vi "host_main(deprecated).vi"() -> ()   [LabVIEW 2023]
uses:
  JSON Command.ctl
  Action.ctl
  <vilib>/FPGAPlugInAG/cRIO-9048/niLvFpga_Open_cRIO-9048.vi
  <vilib>/rvi/interface/common/dynamic/niFpgaDynamicAddResources.vi
  <vilib>/Utility/error.llb/Error Cluster From Error Code.vi
  <vilib>/rvi/errors/niLvFpgaAdjustHostInterfaceError.vi
  <vilib>/rvi/interface/common/niFpgaWaitOnOcc.vi
  <vilib>/FPGAPlugInAG/Dynamic/niLvFpga_Run_Dynamic.vi
  <vilib>/FPGAPlugInAG/Dynamic/niLvFpga_Close_Dynamic.vi
  <vilib>/rvi/interface/nirviOpenFPGA/nirviOpenFPGA.xnode
  FPGA Bitfiles/fpgaproj_FPGATarget_targetmainmem_EQ1ZdgFzOzw.lvbitx
  target_main_mem.vi
  <vilib>/rvi/interface/nirviReadWriteControl/nirviReadWriteControl.xnode
  <vilib>/rvi/interface/nirviMethod/nirviMethod.xnode
  <vilib>/rvi/interface/nirviCloseFPGA/nirviCloseFPGA.xnode
  <vilib>/FPGAPlugInAG/Dynamic/niLvFpga_ConfigureFifo_Dynamic.vi
  <vilib>/rvi/errors/niLvFpgaMergeErrorWithErrorCode.vi
  <vilib>/FPGAPlugInAG/Dynamic/niLvFpga_WriteFifo_Dynamic.vi
  NiFpgaLv.dll
  <vilib>/rvi/interface/Simulation/niFpgaSimulationCallBeginRW.vi
  <vilib>/FPGAPlugInAG/Dynamic/niLvFpga_ReadFifo_Dynamic.vi
  <vilib>/FPGAPlugInAG/Dynamic/niLvFpga_StopFifo_Dynamic.vi
panel:
  out "bytes written":i32
  in  "Stop VI":bool
  out "FPGA VI Reference Out":refnum<k20>
  out "Abort":bool
  out "remote port":u16
  out "remote address":string
  in  "Send PORT":u16=7704
  out "From Client:":string
  out "RAW JSON":T1
  out "ACK sent":string
  out "Laser Toggle 2":bool
  out "Laser Toggle 1":bool
  out "Laser Toggle 0":bool
  in  "Analogue Line 5":u32=10
  in  "Analogue Line 4":u32=10
  in  "Analogue Line 3":u32=10
  out "Digital Line 2":u32
  out "Digital Line 1":u32
  out "Digital Line 0":u32
  out "Analogue Line 2":u8
  out "Analogue Line 1":u8
  out "Analogue Line 0":u8
  in  "FPGA Status Update Loop Time (ms)":u32=1
  out "UDP Sent":string
  in  "Event":string
  in  "Status":string
  in  "Receive PORT":u16=7705
  in  "UDP Address (IP)":string="172.22.11.1"
  out "Boolean array on Host":bool[](array[boolean])
  out "Addr Digital 2":u32
  out "Addr Digital 1":u32
  out "Addr Analogue 1":u32
  out "Addr Analogue 2":u32
  out "Addr Digital 0":u32
  out "Addr Analogue 0":u32
  in  "Digital 2 Action Table":T2[](array[typedef])
  in  "Digital 1 Action Table":T2[](array[typedef])
  in  "Digital 0 Action Table":T2[](array[typedef])
  in  "Analogue 2 Action Table":T2[](array[typedef])
  in  "Analogue 1 Action Table":T2[](array[typedef])
  in  "Analogue 0 Action Table":T2[](array[typedef])
  # "TCP Communication"
  # "Angle, Phase, and Color"
  # "UDP Communication"
  # "Laser On/Off and Power Control"
  # "Action Tables & Experiment Logging"
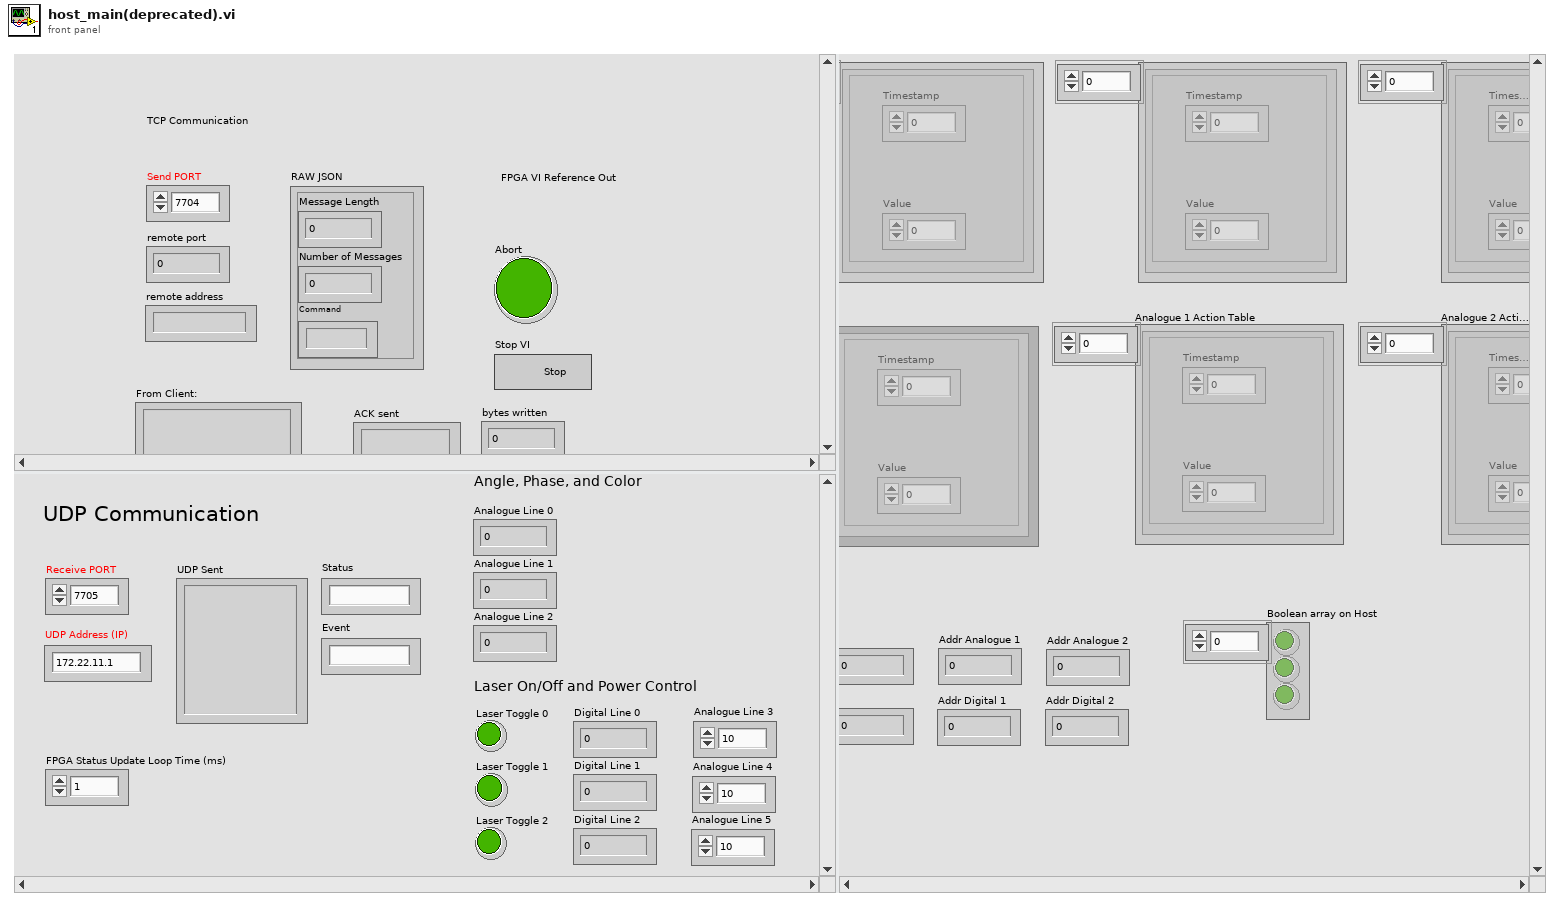
[diagram p1: front panel]
types:
  T1 = typedef "JSON Command.ctl" = cluster{"Message Length":i32, "Number of Messages":i32, "Command":string}
  T2 = typedef "Action.ctl" = cluster{"Timestamp":u32, "Value":u32}
  T3 = cluster{"Digital 2":bool, "Digital 1":bool, "Digital 0":bool}
  T4 = cluster{"Digitals":u8, "Analogue 0":u8, "Analogue 1":u8, "Event":string, "Analogue 2":u8, "Analogue 3":u32, "Analogue 4":u32, "Analogue 5":u32}
  T5 = enum16{"Standard", "Buffered", "CRLF", "Immediate"}
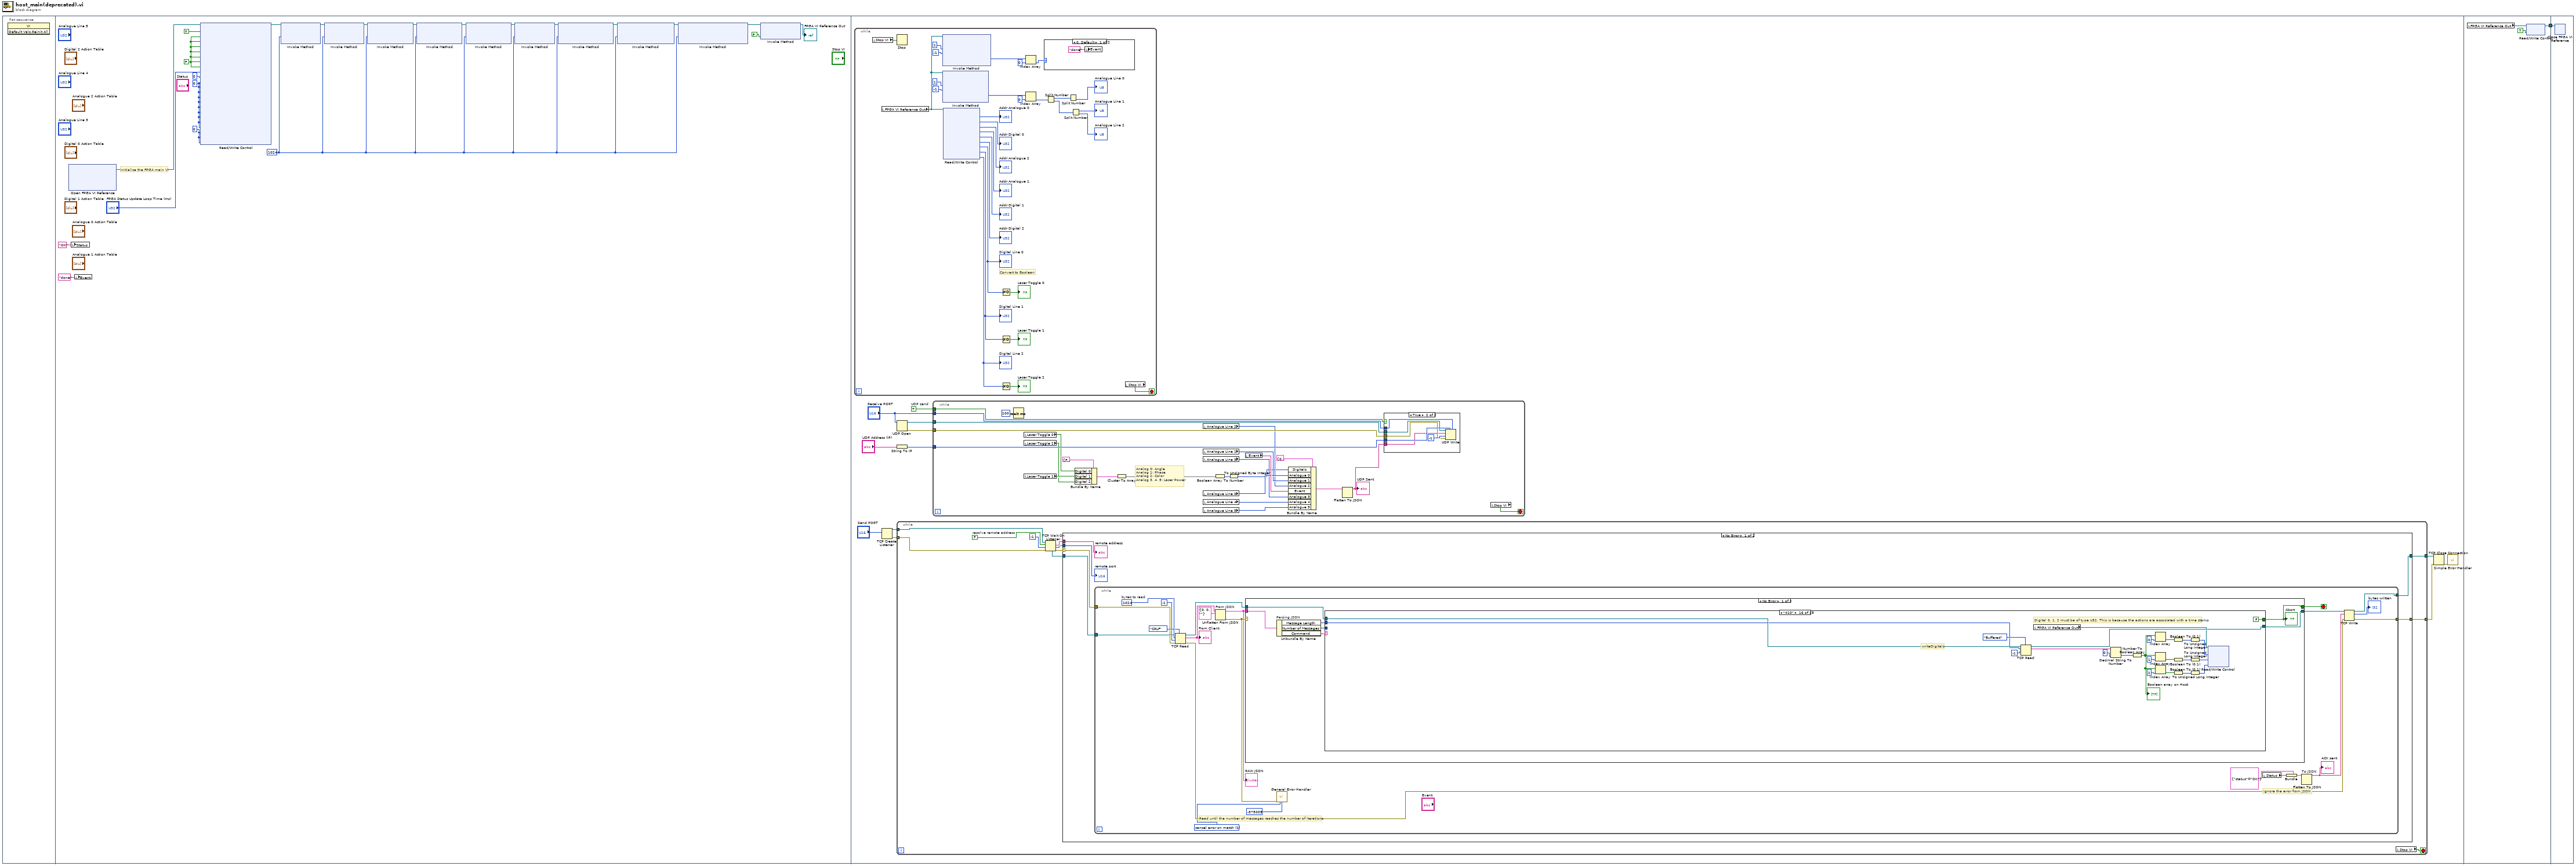
[diagram p0: block diagram]
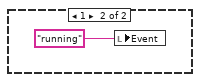
[diagram p2: hidden frame]
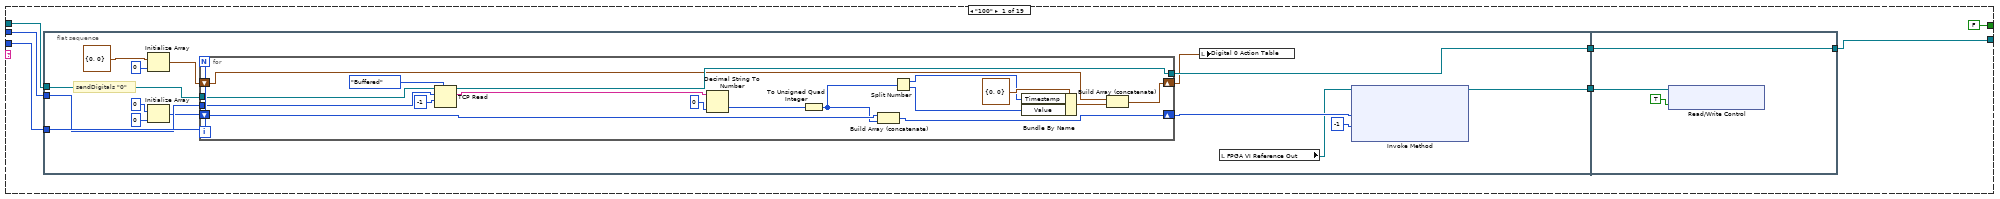
[diagram p4: hidden frame]
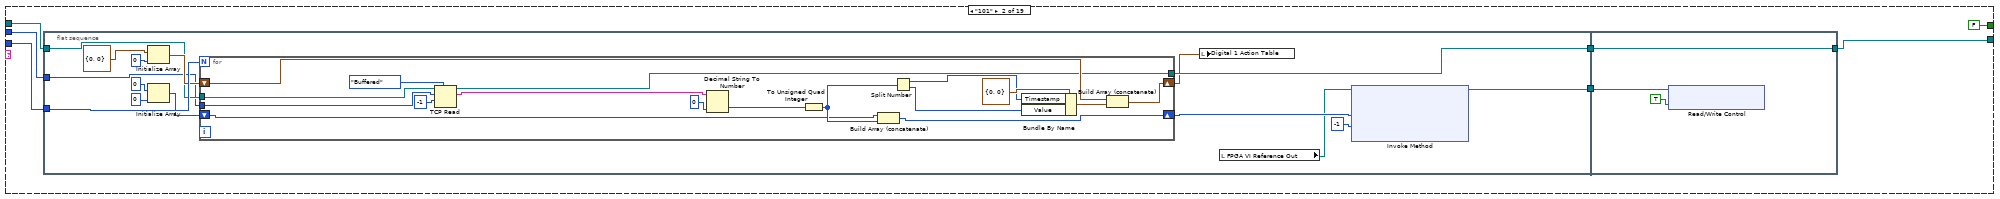
[diagram p5: hidden frame]
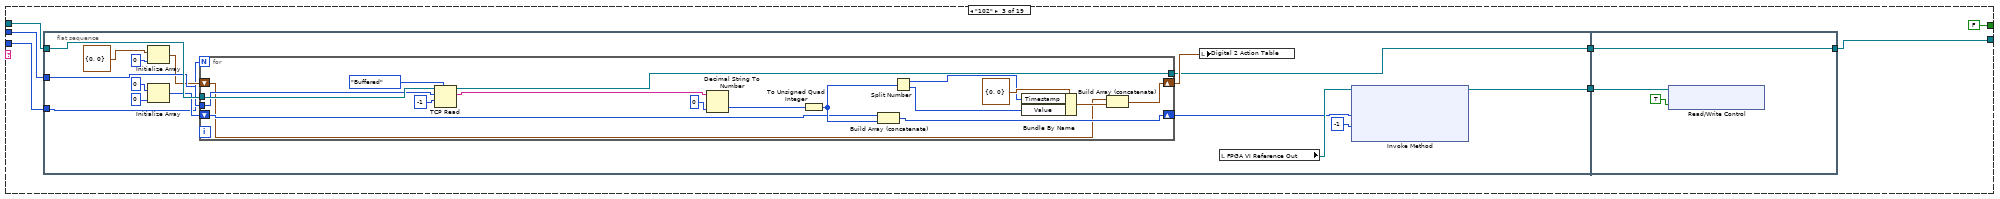
[diagram p6: hidden frame]
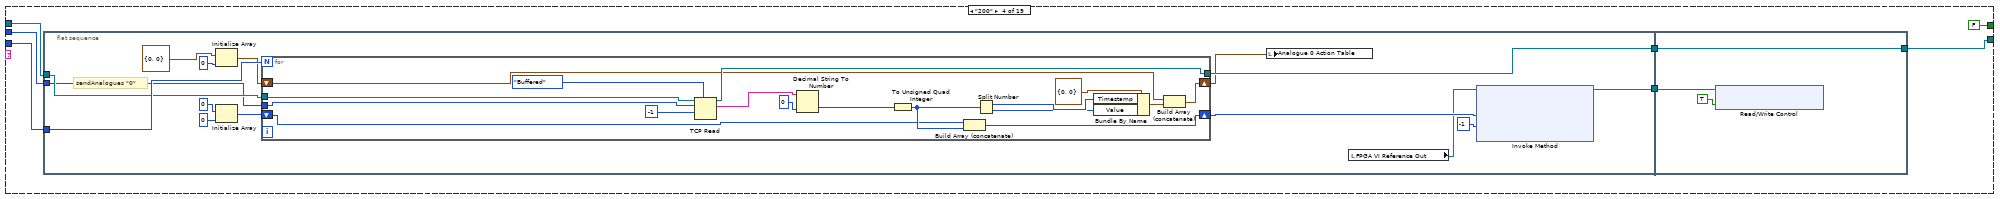
[diagram p7: hidden frame]
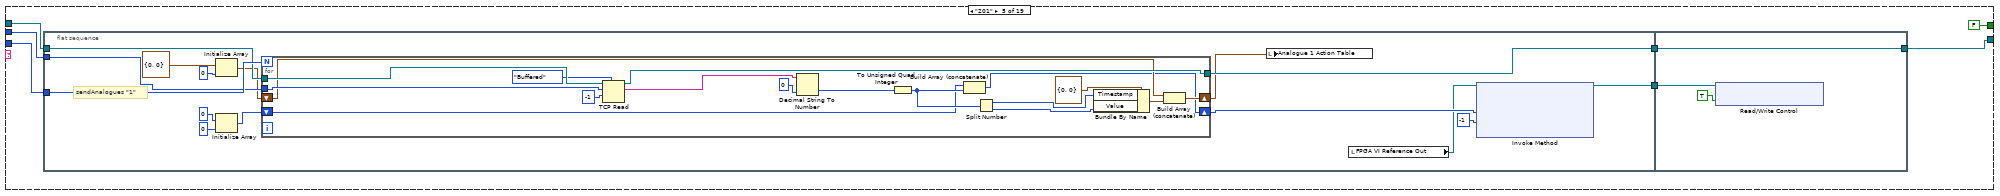
[diagram p8: hidden frame]
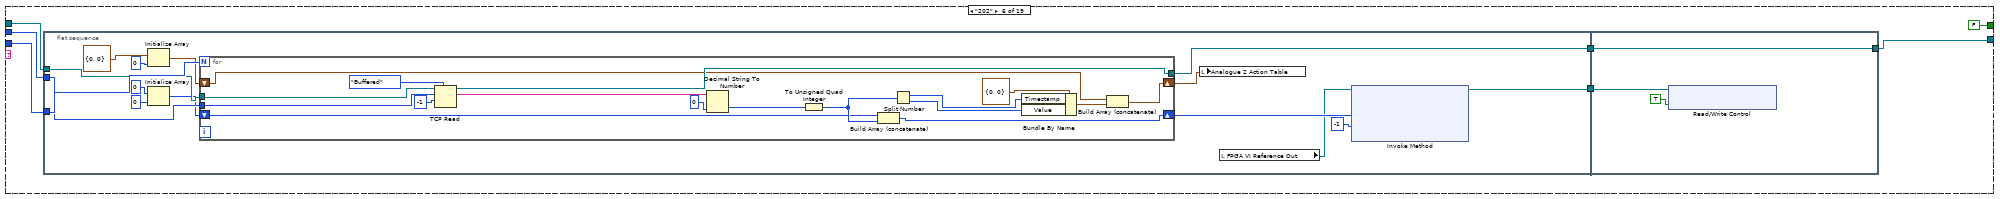
[diagram p9: hidden frame]
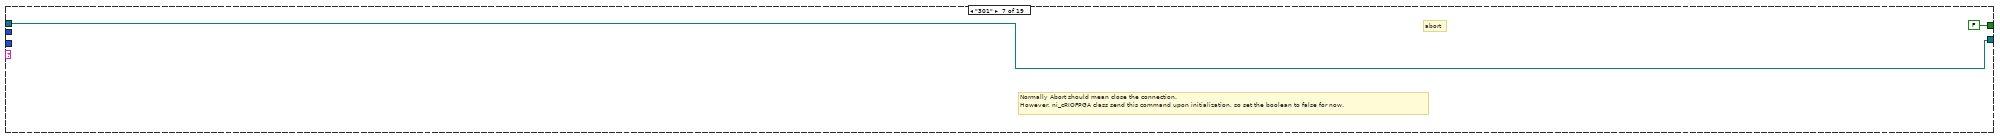
[diagram p10: hidden frame]
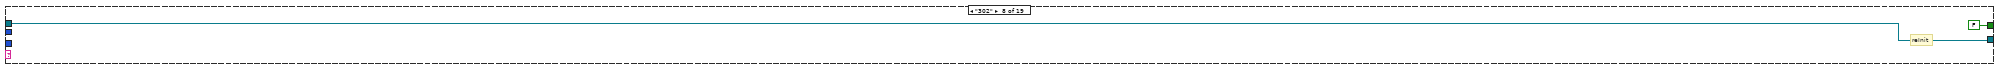
[diagram p11: hidden frame]
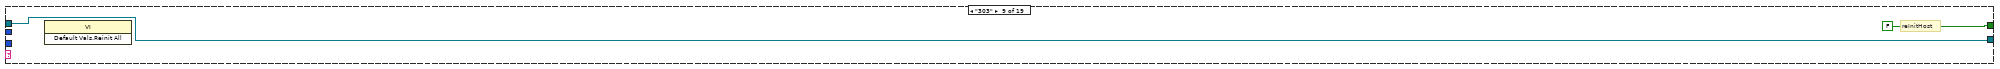
[diagram p12: hidden frame]
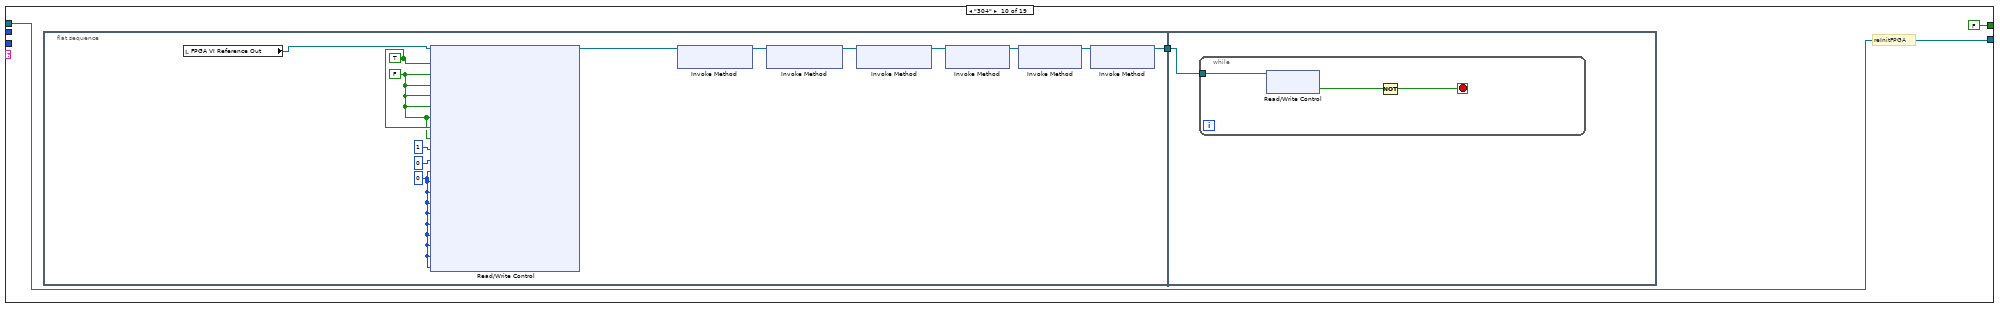
[diagram p13: hidden frame]
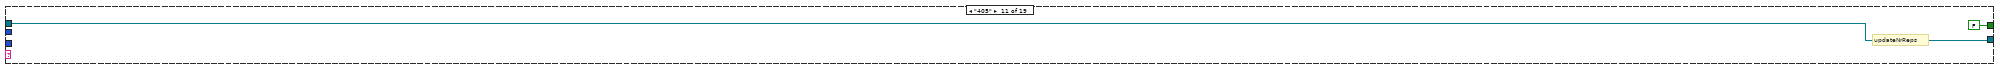
[diagram p14: hidden frame]
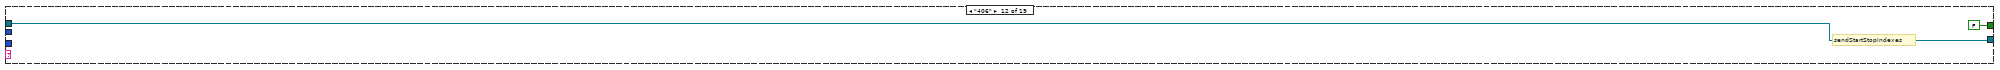
[diagram p15: hidden frame]
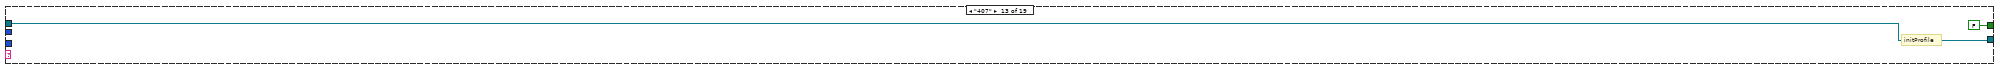
[diagram p16: hidden frame]
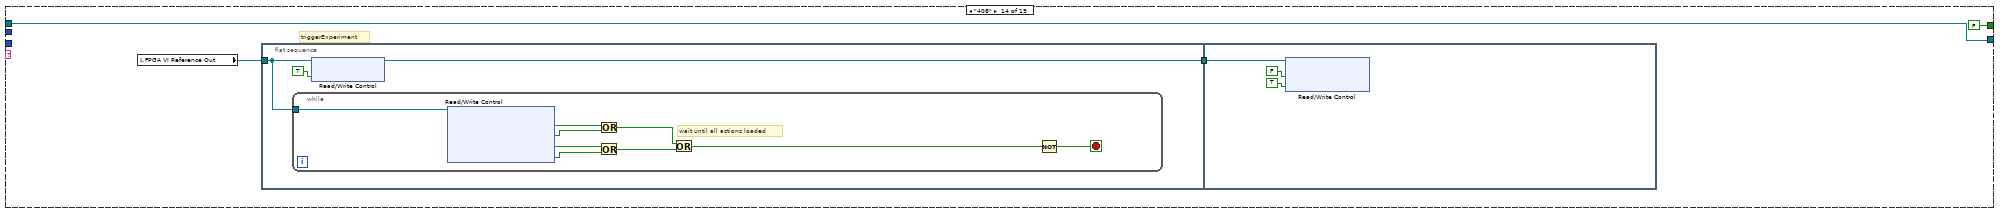
[diagram p17: hidden frame]
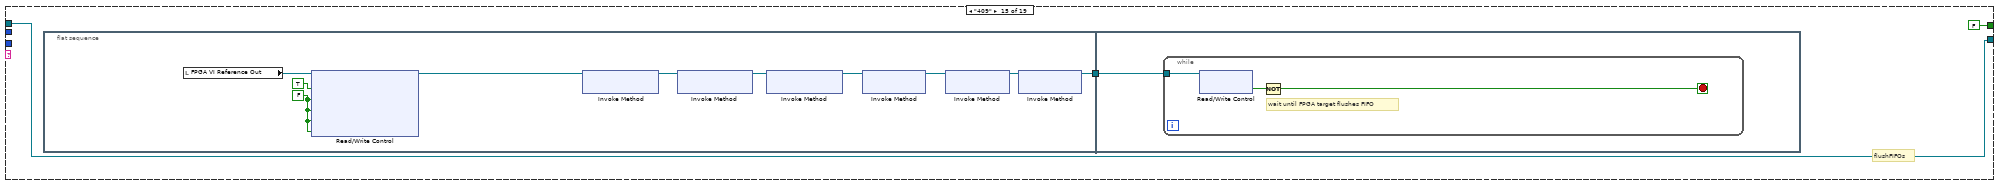
[diagram p18: hidden frame]
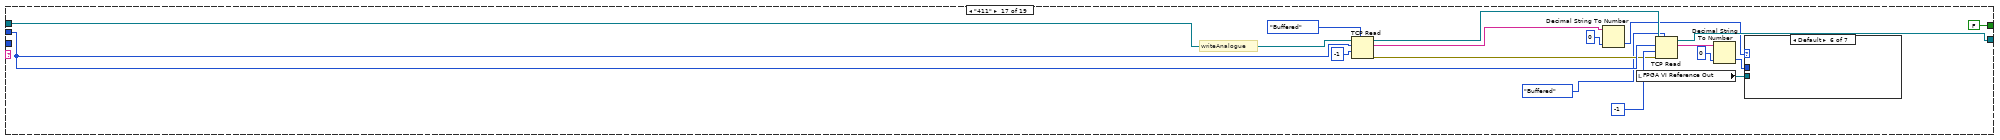
[diagram p19: hidden frame]
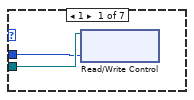
[diagram p20: hidden frame]
diagram:
  n1 = flat-sequence {
    tunnel: [w523] -> w1
    tunnel: w1 -> [w525]
    frame #0 {
      n2 = invoke class="VI" method="Default Vals.Reinit All"() -> ()  [unwired: 3 in, 3 out]
    }
    frame #1 {
      w2 = u32 0 ("Digital 0")
      w3 = u32 0 ("Addr Analogue 0")
      w4 = u32 1024 ("Requested Depth")
      w10 = FALSE ("Action Abort")
      # "Initialize the FPGA main VI"
      n3 = xnode "Open FPGA VI Reference"() -> ("FPGA VI Reference Out"=w11:refnum<k20>)  [unwired: 2 in, 1 out]
      n4 = local write "Status"("OK") -> ()
      n5 = local write "Event"("done") -> ()
      n6 = xnode "Read/Write Control"("FPGA VI Reference In"=w11, "FPGA Tick Reset"=TRUE, "Abort"=w10, "Load Actions Analogue 0"=w10, "Load Actions Analogue 1"=w10, "Load Actions Analogue 2"=w10, "Load Actions Digital 0"=w10, "Flush FIFO"=w10, "Trigger Experiment"=w10, "FPGA Status Update Loop Time (ms)"="FPGA Status Update Loop Time (ms)", "Status Code"=u8 0, "Addr Analogue 0"=w3, "Addr Analogue 1"=w3, "Addr Analogue 2"=w3, "Addr Digital 0"=w3, "Addr Digital 1"=w3, "Addr Digital 2"=w3, "Num of Actions Analogue 0"=w3, "Num of Actions Analogue 1"=w3, "Num of Actions Analogue 2"=w3, "Num of Actions Digital 0"=w3, "Digital 0"=w2, "Digital 1"=w2, "Digital 2"=w2) -> ("FPGA VI Reference Out"=w9:refnum<k20>)  [unwired: 1 in, 1 out]
      n7 = xnode "Invoke Method"("FPGA VI Reference In"=w9, "Requested Depth"=w4) -> ("FPGA VI Reference Out"=w8:refnum<k20>)  [unwired: 1 in, 2 out]
      n8 = xnode "Invoke Method"("FPGA VI Reference In"=w8, "Requested Depth"=w4) -> ("FPGA VI Reference Out"=w7:refnum<k20>)  [unwired: 1 in, 2 out]
      n9 = xnode "Invoke Method"("FPGA VI Reference In"=w7, "Requested Depth"=w4) -> ("FPGA VI Reference Out"=w22:refnum<k20>)  [unwired: 1 in, 2 out]
      n10 = xnode "Invoke Method"("FPGA VI Reference In"=w22, "Requested Depth"=w4) -> ("FPGA VI Reference Out"=w12:refnum<k20>)  [unwired: 1 in, 2 out]
      n11 = xnode "Invoke Method"("FPGA VI Reference In"=w12, "Requested Depth"=w4) -> ("FPGA VI Reference Out"=w21:refnum<k20>)  [unwired: 1 in, 2 out]
      n12 = xnode "Invoke Method"("FPGA VI Reference In"=w21, "Requested Depth"=w4) -> ("FPGA VI Reference Out"=w20:refnum<k20>)  [unwired: 1 in, 2 out]
      n13 = xnode "Invoke Method"("FPGA VI Reference In"=w20, "Requested Depth"=w4) -> ("FPGA VI Reference Out"=w19:refnum<k20>)  [unwired: 1 in, 2 out]
      n14 = xnode "Invoke Method"("FPGA VI Reference In"=w19, "Requested Depth"=w4) -> ("FPGA VI Reference Out"=w6:refnum<k20>)  [unwired: 1 in, 2 out]
      n15 = xnode "Invoke Method"("FPGA VI Reference In"=w6, "Requested Depth"=w4) -> ("FPGA VI Reference Out"=w5:refnum<k20>)  [unwired: 1 in, 2 out]
      n16 = xnode "Invoke Method"("FPGA VI Reference In"=w5, "Wait Until Done (F)"=FALSE) -> ("FPGA VI Reference Out"=→"FPGA VI Reference Out":refnum<k20>)  [unwired: 1 in, 1 out]
    }
    frame #2 {
      w24 = TRUE  # UDP send
      n17 = while {
        stop <- w50 stop-if-true
        # "Convert to Boolean"
        n18 = local read "Stop VI"() -> (w49:bool)
        n19 = local read "FPGA VI Reference Out"() -> (w42:refnum<k20>)
        n20 = Stop(stop? (T)=w49) -> ()
        n21 = xnode "Invoke Method"("FPGA VI Reference In"=w42, "Number of Elements"=u32 1, "Timeout (ms)"=-1) -> ("Data"=w54:u8[])  [unwired: 1 in, 3 out]
        n22 = xnode "Invoke Method"("FPGA VI Reference In"=w42, "Number of Elements"=u32 1, "Timeout (ms)"=-1) -> ("Data"=w63:u32[])  [unwired: 1 in, 3 out]
        n23 = xnode "Read/Write Control"("FPGA VI Reference In"=w42) -> ("Addr Analogue 0"=→"Addr Analogue 0":u32, "Addr Digital 0"=→"Addr Digital 0":u32, "Addr Analogue 2"=→"Addr Analogue 2":u32, "Addr Analogue 1"=→"Addr Analogue 1":u32, "Addr Digital 1"=→"Addr Digital 1":u32, "Addr Digital 2"=→"Addr Digital 2":u32, "Digital 0"=w36:u32, "Digital 1"=w37:u32, "Digital 2"=w38:u32)  [unwired: 1 in, 2 out]
        "Digital Line 0" <- w36
        "Digital Line 1" <- w37
        "Digital Line 2" <- w38
        n24 = Not Equal To 0?(x=w36) -> (x != 0?=→"Laser Toggle 0":bool)
        n25 = Not Equal To 0?(x=w37) -> (x != 0?=→"Laser Toggle 1":bool)
        n26 = Not Equal To 0?(x=w38) -> (x != 0?=→"Laser Toggle 2":bool)
        n27 = Index Array(array=w54, index=0) -> (element=w55:u8)
        n28 = Index Array(array=w63, index=0) -> (element=w61:u32)
        n29 = case shown="0, Default" w55 {
          frame 0, Default {
            n30 = local write "Event"("done") -> ()
          }
          frame 1 {
            n31 = local write "Event"("running") -> ()
          }
        }
        n32 = Split Number(x=w61) -> (hi(x)=w60:u16, lo(x)=w59:u16)
        n33 = Split Number(x=w60) -> (lo(x)=→"Analogue Line 0":u8)  [unwired: 1 out]
        n34 = Split Number(x=w59) -> (hi(x)=→"Analogue Line 1":u8, lo(x)=→"Analogue Line 2":u8)
        n35 = local read "Stop VI"() -> (w50:bool)
      }
      n36 = TCP Create Listener(10:"Send PORT") -> (0:w33:errorcluster, 3:w32:refnum<k5>)  [unwired: 4 in, 1 out]
      n37 = UDP Open(11:"Receive PORT") -> (port=w27:refnum<k16>, 0:w29:errorcluster)  [unwired: 4 in, 1 out]
      n38 = String To IP(1:"UDP Address (IP)") -> (0:w26:u32)
      n39 = while {
        tunnel: w32 -> [w109]
        tunnel: w33 -> [w108]
        tunnel: [w107] -> w34
        tunnel: [w106] -> w35
        stop <- w99 stop-if-true
        w103 = FALSE  # resolve remote address
        n40 = TCP Wait On Listener(8:w108, 9:-1 ("timeout ms (wait forever: -1)"), 10:w103, 11:w109) -> (0:w104:errorcluster, 1:w101:u16, 2:w102:string, 4:w100:refnum<k5>)  [unwired: 1 out]
        n41 = case shown="No Error" w104 {
          selector: w104 -> [w112 w520]
          tunnel: w100 -> [w115 w521]
          tunnel: [w114 w520] -> w107
          tunnel: [w113 w521] -> w106
          tunnel: w102 -> [w110 _]
          tunnel: w101 -> [w111 _]
          frame No Error {
            n42 = while {
              tunnel: w112 -> [w127]
              tunnel: [w129] -> w114
              tunnel: w115 -> [w130]
              tunnel: [w128] -> w113
              stop <- w121 stop-if-true
              w125 = 1 items=["no exception", "cancel error on match", "set error on match"] ("[exception action] (none:0)")
              w136 = 1024  # bytes to read
              # "Ignore the error from JSON"
              # "Read until the number of messages reaches the number of iterations"
              n43 = TCP Read(connection ID=w130, bytes to read=w136, error in (no error)=w127, 7:T5."CRLF" ("mode (standard)"), 9:-1 ("timeout ms (25000)")) -> (connection ID out=w119:refnum<k5>, data out=w133:string, error out=w137:errorcluster)
              "From Client:" <- w133
              n44 = Unflatten From JSON "From JSON"(JSON string=w133, type and defaults=T1 {"Message Length"=0, "Number of Messages"=0, "Command"=""} ("JSON Command")) -> (value=w122:T1, error out=w123:errorcluster)  [unwired: 5 in]
              "RAW JSON" <- w122
              n45 = case shown="No Error" w123 {
                tunnel: w122 -> [w144 _]
                tunnel: [w142 TRUE] -> w121
                tunnel: w119 -> [w140 w518]
                tunnel: [w139 w518] -> w118
                frame No Error {
                  n46 = Unbundle By Name "Parsing JSON"(w144) -> ("Message Length"=w138:i32, "Number of Messages"=w141:i32, "Command"=w143:string)
                  n47 = case shown="\"410\"" w143 {
                    tunnel: [FALSE FALSE FALSE FALSE FALSE FALSE FALSE FALSE FALSE FALSE FALSE FALSE FALSE FALSE FALSE FALSE FALSE FALSE TRUE] -> w142
                    tunnel: w141 -> [w150 w193 w229 w276 w319 w360 _ _ _ _ _ _ _ _ _ _ _ _ _]
                    tunnel: w140 -> [w149 w192 w235 w275 w317 w359 w397 w399 w401 w404 w423 w425 w427 w431 w449 w486 w501 w514 w517]
                    tunnel: [w148 w190 w233 w274 w316 w357 w397 w399 w401 w404 w423 w425 w427 w431 w449 w485 w492 w514 w517] -> w139
                    tunnel: w138 -> [w147 w191 w234 w273 w315 w358 _ _ _ _ _ _ _ _ _ w483 w497 _ _]
                    frame "100" {
                      n48 = flat-sequence {
                        tunnel: w150 -> [w166]
                        tunnel: w149 -> [w165]
                        tunnel: w147 -> [w163]
                        tunnel: [w164] -> w146
                        tunnel: [w152] -> w145
                        tunnel: [w186] -> w148
                        tunnel: w146 -> [w186]
                        tunnel: w145 -> [w185]
                        frame #0 {
                          # "sendDigitals \"0\""
                          n49 = Initialize Array(T2 {"Timestamp"=0, "Value"=0} ("Action"), 0 ("dimension size")) -> (w158:T2[])
                          n50 = Initialize Array(u64 0 ("element"), 0 ("dimension size")) -> (w157:u64[])
                          n51 = for {
                            N: w166 -> [_]
                            tunnel: w165 -> [w182]
                            tunnel: [w181] -> w164
                            tunnel: w163 -> [w180]
                            shift-right: [w168] -> w155
                            shift-left: w157 -> [w170]
                            shift-right: [w171] -> w156
                            shift-left: w158 -> [w173]
                            n52 = TCP Read(connection ID=w182, bytes to read=w180, 7:T5."Buffered" ("mode (standard)"), 9:-1 ("timeout ms (25000)")) -> (connection ID out=w181:refnum<k5>, data out=w177:string)  [unwired: 1 in, 1 out]
                            n53 = Decimal String To Number(string=w177, default (0L)=u64 0 ("default (0 I32)")) -> (number=w178:u64)  [unwired: 1 in, 1 out]
                            n54 = To Unsigned Quad Integer(1:w178) -> (0:w169:u64)
                            n55 = Build Array (concatenate)(w170, w169) -> (w168:u64[])
                            n56 = Split Number(x=w169) -> (hi(x)=w175:u32, lo(x)=w174:u32)
                            n57 = Bundle By Name(cluster=T2 {"Timestamp"=0, "Value"=0} ("Action"), "Timestamp"=w175, "Value"=w174) -> (w172:T2)
                            n58 = Build Array (concatenate)(w173, w172) -> (w171:T2[])
                          }
                          n59 = local write "Digital 0 Action Table"(w156) -> ()
                          n60 = local read "FPGA VI Reference Out"() -> (w153:refnum<k20>)
                          n61 = xnode "Invoke Method"("FPGA VI Reference In"=w153, "Data"=w155, "Timeout (ms)"=-1) -> ("FPGA VI Reference Out"=w152:refnum<k20>)  [unwired: 1 in, 2 out]
                        }
                        frame #1 {
                          n62 = xnode "Read/Write Control"("FPGA VI Reference In"=w185, "Load Actions Digital 0"=TRUE ("Load Actions")) -> ()  [unwired: 1 in, 2 out]
                        }
                      }
                    }
                    frame "101" {
                      n63 = flat-sequence {
                        tunnel: w193 -> [w204]
                        tunnel: w192 -> [w201]
                        tunnel: w191 -> [w200]
                        tunnel: [w199] -> w189
                        tunnel: [w194] -> w188
                        tunnel: [w228] -> w190
                        tunnel: w189 -> [w228]
                        tunnel: w188 -> [w227]
                        frame #0 {
                          n64 = Initialize Array(T2 {"Timestamp"=0, "Value"=0} ("Action"), 0 ("dimension size")) -> (w202:T2[])
                          n65 = Initialize Array(u64 0 ("element"), 0 ("dimension size")) -> (w203:u64[])
                          n66 = for {
                            N: w204 -> [_]
                            shift-right: [w213] -> w198
                            shift-left: w202 -> [w214]
                            shift-right: [w210] -> w197
                            shift-left: w203 -> [w211]
                            tunnel: w201 -> [w224]
                            tunnel: w200 -> [w223]
                            tunnel: [w209] -> w199
                            n67 = TCP Read(connection ID=w224, bytes to read=w223, 7:T5."Buffered" ("mode (standard)"), 9:-1 ("timeout ms (25000)")) -> (connection ID out=w209:refnum<k5>, data out=w221:string)  [unwired: 1 in, 1 out]
                            n68 = Decimal String To Number(string=w221, default (0L)=u64 0 ("default (0 I32)")) -> (number=w219:u64)  [unwired: 1 in, 1 out]
                            n69 = To Unsigned Quad Integer(1:w219) -> (0:w212:u64)
                            n70 = Build Array (concatenate)(w211, w212) -> (w210:u64[])
                            n71 = Split Number(x=w212) -> (hi(x)=w217:u32, lo(x)=w216:u32)
                            n72 = Bundle By Name(cluster=T2 {"Timestamp"=0, "Value"=0} ("Action"), "Timestamp"=w217, "Value"=w216) -> (w215:T2)
                            n73 = Build Array (concatenate)(w214, w215) -> (w213:T2[])
                          }
                          n74 = local write "Digital 1 Action Table"(w198) -> ()
                          n75 = local read "FPGA VI Reference Out"() -> (w195:refnum<k20>)
                          n76 = xnode "Invoke Method"("FPGA VI Reference In"=w195, "Data"=w197, "Timeout (ms)"=-1) -> ("FPGA VI Reference Out"=w194:refnum<k20>)  [unwired: 1 in, 2 out]
                        }
                        frame #1 {
                          n77 = xnode "Read/Write Control"("FPGA VI Reference In"=w227, "Load Actions Digital 1"=TRUE) -> ()  [unwired: 1 in, 2 out]
                        }
                      }
                    }
                    frame "102" {
                      n78 = flat-sequence {
                        tunnel: w235 -> [w246]
                        tunnel: w234 -> [w245]
                        tunnel: [w238] -> w232
                        tunnel: [w237] -> w230
                        tunnel: w229 -> [w236]
                        tunnel: [w270] -> w233
                        tunnel: w232 -> [w270]
                        tunnel: w230 -> [w269]
                        frame #0 {
                          n79 = Initialize Array(T2 {"Timestamp"=0, "Value"=0} ("Action"), 0 ("dimension size")) -> (w244:T2[])
                          n80 = Initialize Array(u64 0 ("element"), 0 ("dimension size")) -> (w243:u64[])
                          n81 = for {
                            N: w236 -> [_]
                            tunnel: w246 -> [w266]
                            tunnel: w245 -> [w265]
                            shift-right: [w255] -> w240
                            shift-left: w243 -> [w256]
                            shift-right: [w252] -> w242
                            shift-left: w244 -> [w253]
                            tunnel: [w251] -> w238
                            n82 = TCP Read(connection ID=w266, bytes to read=w265, 7:T5."Buffered" ("mode (standard)"), 9:-1 ("timeout ms (25000)")) -> (connection ID out=w251:refnum<k5>, data out=w262:string)  [unwired: 1 in, 1 out]
                            n83 = Decimal String To Number(string=w262, default (0L)=u64 0 ("default (0 I32)")) -> (number=w261:u64)  [unwired: 1 in, 1 out]
                            n84 = To Unsigned Quad Integer(1:w261) -> (0:w257:u64)
                            n85 = Build Array (concatenate)(w256, w257) -> (w255:u64[])
                            n86 = Split Number(x=w257) -> (hi(x)=w259:u32, lo(x)=w258:u32)
                            n87 = Bundle By Name(cluster=T2 {"Timestamp"=0, "Value"=0} ("Action"), "Timestamp"=w259, "Value"=w258) -> (w254:T2)
                            n88 = Build Array (concatenate)(w253, w254) -> (w252:T2[])
                          }
                          n89 = local write "Digital 2 Action Table"(w242) -> ()
                          n90 = local read "FPGA VI Reference Out"() -> (w241:refnum<k20>)
                          n91 = xnode "Invoke Method"("FPGA VI Reference In"=w241, "Data"=w240, "Timeout (ms)"=-1) -> ("FPGA VI Reference Out"=w237:refnum<k20>)  [unwired: 1 in, 2 out]
                        }
                        frame #1 {
                          n92 = xnode "Read/Write Control"("FPGA VI Reference In"=w269, "Load Actions Digital 2"=TRUE) -> ()  [unwired: 1 in, 2 out]
                        }
                      }
                    }
                    frame "200" {
                      n93 = flat-sequence {
                        tunnel: w276 -> [w292]
                        tunnel: w275 -> [w291]
                        tunnel: w273 -> [w289]
                        tunnel: [w290] -> w272
                        tunnel: [w278] -> w271
                        tunnel: [w312] -> w274
                        tunnel: w272 -> [w312]
                        tunnel: w271 -> [w311]
                        frame #0 {
                          # "sendAnalogues \"0\""
                          n94 = Initialize Array(T2 {"Timestamp"=0, "Value"=0} ("Action"), 0 ("dimension size")) -> (w286:T2[])
                          n95 = Initialize Array(u64 0 ("element"), 0 ("dimension size")) -> (w282:u64[])
                          n96 = for {
                            N: w292 -> [_]
                            tunnel: w291 -> [w308]
                            tunnel: [w306] -> w290
                            tunnel: w289 -> [w305]
                            shift-right: [w296] -> w285
                            shift-left: w286 -> [w301]
                            shift-right: [w293] -> w281
                            shift-left: w282 -> [w294]
                            n97 = TCP Read(connection ID=w308, bytes to read=w305, 7:T5."Buffered" ("mode (standard)"), 9:-1 ("timeout ms (25000)")) -> (connection ID out=w306:refnum<k5>, data out=w303:string)  [unwired: 1 in, 1 out]
                            n98 = Decimal String To Number(string=w303, default (0L)=u64 0) -> (number=w304:u64)  [unwired: 1 in, 1 out]
                            n99 = To Unsigned Quad Integer(1:w304) -> (0:w295:u64)
                            n100 = Build Array (concatenate)(w294, w295) -> (w293:u64[])
                            n101 = Split Number(x=w295) -> (hi(x)=w299:u32, lo(x)=w298:u32)
                            n102 = Bundle By Name(cluster=T2 {"Timestamp"=0, "Value"=0} ("Action"), "Timestamp"=w299, "Value"=w298) -> (w297:T2)
                            n103 = Build Array (concatenate)(w301, w297) -> (w296:T2[])
                          }
                          n104 = local write "Analogue 0 Action Table"(w285) -> ()
                          n105 = local read "FPGA VI Reference Out"() -> (w279:refnum<k20>)
                          n106 = xnode "Invoke Method"("FPGA VI Reference In"=w279, "Data"=w281, "Timeout (ms)"=-1) -> ("FPGA VI Reference Out"=w278:refnum<k20>)  [unwired: 1 in, 2 out]
                        }
                        frame #1 {
                          n107 = xnode "Read/Write Control"("FPGA VI Reference In"=w311, "Load Actions Analogue 0"=TRUE ("Load Actions")) -> ()  [unwired: 1 in, 2 out]
                        }
                      }
                    }
                    frame "201" {
                      n108 = flat-sequence {
                        tunnel: w319 -> [w334]
                        tunnel: w317 -> [w333]
                        tunnel: w315 -> [w331]
                        tunnel: [w332] -> w314
                        tunnel: [w320] -> w313
                        tunnel: [w354] -> w316
                        tunnel: w314 -> [w354]
                        tunnel: w313 -> [w353]
                        frame #0 {
                          # "sendAnalogues \"1\""
                          n109 = Initialize Array(T2 {"Timestamp"=0, "Value"=0} ("Action"), 0 ("dimension size")) -> (w328:T2[])
                          n110 = Initialize Array(u64 0, 0 ("dimension size")) -> (w323:u64[])
                          n111 = for {
                            N: w334 -> [_]
                            tunnel: w333 -> [w351]
                            tunnel: [w350] -> w332
                            tunnel: w331 -> [w349]
                            shift-right: [w340] -> w326
                            shift-left: w328 -> [w341]
                            shift-right: [w337] -> w322
                            shift-left: w323 -> [w338]
                            n112 = TCP Read(connection ID=w351, bytes to read=w349, 7:T5."Buffered" ("mode (standard)"), 9:-1 ("timeout ms (25000)")) -> (connection ID out=w350:refnum<k5>, data out=w346:string)  [unwired: 1 in, 1 out]
                            n113 = Decimal String To Number(string=w346, default (0L)=u64 0 ("default (0 I32)")) -> (number=w345:u64)  [unwired: 1 in, 1 out]
                            n114 = To Unsigned Quad Integer(1:w345) -> (0:w339:u64)
                            n115 = Build Array (concatenate)(w338, w339) -> (w337:u64[])
                            n116 = Split Number(x=w339) -> (hi(x)=w336:u32, lo(x)=w344:u32)
                            n117 = Bundle By Name(cluster=T2 {"Timestamp"=0, "Value"=0} ("Action"), "Timestamp"=w336, "Value"=w344) -> (w342:T2)
                            n118 = Build Array (concatenate)(w341, w342) -> (w340:T2[])
                          }
                          n119 = local write "Analogue 1 Action Table"(w326) -> ()
                          n120 = local read "FPGA VI Reference Out"() -> (w321:refnum<k20>)
                          n121 = xnode "Invoke Method"("FPGA VI Reference In"=w321, "Data"=w322, "Timeout (ms)"=-1) -> ("FPGA VI Reference Out"=w320:refnum<k20>)  [unwired: 1 in, 2 out]
                        }
                        frame #1 {
                          n122 = xnode "Read/Write Control"("FPGA VI Reference In"=w353, "Load Actions Analogue 1"=TRUE ("Load Actions")) -> ()  [unwired: 1 in, 2 out]
                        }
                      }
                    }
                    frame "202" {
                      n123 = flat-sequence {
                        tunnel: w360 -> [w376]
                        tunnel: w359 -> [w371]
                        tunnel: w358 -> [w370]
                        tunnel: [w369] -> w356
                        tunnel: [w363] -> w355
                        tunnel: [w396] -> w357
                        tunnel: w356 -> [w396]
                        tunnel: w355 -> [w395]
                        frame #0 {
                          n124 = Initialize Array(T2 {"Timestamp"=0, "Value"=0} ("Action"), 0 ("dimension size")) -> (w368:T2[])
                          n125 = Initialize Array(u64 0 ("element"), 0 ("dimension size")) -> (w366:u64[])
                          n126 = for {
                            N: w376 -> [_]
                            tunnel: w371 -> [w392]
                            tunnel: w370 -> [w391]
                            tunnel: [w388] -> w369
                            shift-right: [w381] -> w367
                            shift-left: w368 -> [w382]
                            shift-right: [w378] -> w365
                            shift-left: w366 -> [w379]
                            n127 = TCP Read(connection ID=w392, bytes to read=w391, 7:T5."Buffered" ("mode (standard)"), 9:-1 ("timeout ms (25000)")) -> (connection ID out=w388:refnum<k5>, data out=w389:string)  [unwired: 1 in, 1 out]
                            n128 = Decimal String To Number(string=w389, default (0L)=u64 0 ("default (0 I32)")) -> (number=w387:u64)  [unwired: 1 in, 1 out]
                            n129 = To Unsigned Quad Integer(1:w387) -> (0:w380:u64)
                            n130 = Build Array (concatenate)(w379, w380) -> (w378:u64[])
                            n131 = Split Number(x=w380) -> (hi(x)=w385:u32, lo(x)=w384:u32)
                            n132 = Bundle By Name(cluster=T2 {"Timestamp"=0, "Value"=0} ("Action"), "Timestamp"=w385, "Value"=w384) -> (w383:T2)
                            n133 = Build Array (concatenate)(w382, w383) -> (w381:T2[])
                          }
                          n134 = local write "Analogue 2 Action Table"(w367) -> ()
                          n135 = local read "FPGA VI Reference Out"() -> (w362:refnum<k20>)
                          n136 = xnode "Invoke Method"("FPGA VI Reference In"=w362, "Data"=w365, "Timeout (ms)"=-1) -> ("FPGA VI Reference Out"=w363:refnum<k20>)  [unwired: 1 in, 2 out]
                        }
                        frame #1 {
                          n137 = xnode "Read/Write Control"("FPGA VI Reference In"=w395, "Load Actions Analogue 2"=TRUE ("Load Actions")) -> ()  [unwired: 1 in, 2 out]
                        }
                      }
                    }
                    frame "301" {
                      # "Normally Abort should mean close the connection.\nHowever, ni_cRIOFPGA class send this command upon initialization, so set the boolean to false for now."
                      # "abort"
                    }
                    frame "302" {
                      # "reInit"
                    }
                    frame "303" {
                      # "reInitHost"
                      n138 = invoke class="VI" method="Default Vals.Reinit All"() -> ()  [unwired: 3 in, 3 out]
                    }
                    frame "304" {
                      # "reInitFPGA"
                      n139 = flat-sequence {
                        tunnel: [w406] -> w403
                        tunnel: w403 -> [w419]
                        frame #0 {
                          w413 = u32 0 ("Addr Analogue 0")
                          w416 = FALSE ("Abort")
                          w417 = TRUE ("FPGA Tick Reset")
                          n140 = local read "FPGA VI Reference Out"() -> (w418:refnum<k20>)
                          n141 = xnode "Read/Write Control"("FPGA VI Reference In"=w418, "FPGA Tick Reset"=w417, "Abort"=w416, "Load Actions Analogue 0"=w416, "Load Actions Analogue 1"=w416, "Load Actions Analogue 2"=w416, "Load Actions Digital 0"=w416, "Flush FIFO"=w417, "Trigger Experiment"=w416, "FPGA Status Update Loop Time (ms)"=u32 1, "Status Code"=u8 0, "Addr Analogue 0"=w413, "Addr Analogue 1"=w413, "Addr Analogue 2"=w413, "Addr Digital 0"=w413, "Addr Digital 1"=w413, "Addr Digital 2"=w413, "Num of Actions Analogue 0"=w413, "Num of Actions Analogue 1"=w413, "Num of Actions Analogue 2"=w413, "Num of Actions Digital 0"=w413) -> ("FPGA VI Reference Out"=w407:refnum<k20>)  [unwired: 1 in, 1 out]
                          n142 = xnode "Invoke Method"("FPGA VI Reference In"=w407) -> ("FPGA VI Reference Out"=w412:refnum<k20>)  [unwired: 1 in, 1 out]
                          n143 = xnode "Invoke Method"("FPGA VI Reference In"=w412) -> ("FPGA VI Reference Out"=w411:refnum<k20>)  [unwired: 1 in, 1 out]
                          n144 = xnode "Invoke Method"("FPGA VI Reference In"=w411) -> ("FPGA VI Reference Out"=w410:refnum<k20>)  [unwired: 1 in, 1 out]
                          n145 = xnode "Invoke Method"("FPGA VI Reference In"=w410) -> ("FPGA VI Reference Out"=w409:refnum<k20>)  [unwired: 1 in, 1 out]
                          n146 = xnode "Invoke Method"("FPGA VI Reference In"=w409) -> ("FPGA VI Reference Out"=w408:refnum<k20>)  [unwired: 1 in, 1 out]
                          n147 = xnode "Invoke Method"("FPGA VI Reference In"=w408) -> ("FPGA VI Reference Out"=w406:refnum<k20>)  [unwired: 1 in, 1 out]
                        }
                        frame #1 {
                          n148 = while {
                            tunnel: w419 -> [w422]
                            stop <- w420 stop-if-true
                            n149 = xnode "Read/Write Control"("FPGA VI Reference In"=w422) -> ("Flush FIFO"=w421:bool)  [unwired: 1 in, 2 out]
                            n150 = Not(x=w421) -> (.not. x?=w420:bool)
                          }
                        }
                      }
                    }
                    frame "405" {
                      # "updateNrReps"
                    }
                    frame "406" {
                      # "sendStartStopIndexes"
                    }
                    frame "407" {
                      # "initProfile"
                    }
                    frame "408" {
                      # "triggerExperiment"
                      n151 = local read "FPGA VI Reference Out"() -> (w430:refnum<k20>)
                      n152 = flat-sequence {
                        tunnel: w430 -> [w433]
                        tunnel: [w435] -> w429
                        tunnel: w429 -> [w447]
                        frame #0 {
                          n153 = while {
                            tunnel: w433 -> [w444]
                            stop <- w443 stop-if-true
                            # "wait until all actions loaded"
                            n154 = xnode "Read/Write Control"("FPGA VI Reference In"=w444) -> ("Load Actions Analogue 0"=w439:bool, "Load Actions Analogue 1"=w438:bool, "Load Actions Analogue 2"=w437:bool, "Load Actions Analogue 2"=w436:bool)  [unwired: 1 in, 2 out]
                            n155 = Or(x=w439, y=w438) -> (x .or. y?=w441:bool)
                            n156 = Or(x=w437, y=w436) -> (x .or. y?=w440:bool)
                            n157 = Or(x=w441, y=w440) -> (x .or. y?=w442:bool)
                            n158 = Not(x=w442) -> (.not. x?=w443:bool)
                          }
                          n159 = xnode "Read/Write Control"("FPGA VI Reference In"=w433, "FPGA Tick Reset"=TRUE) -> ("FPGA VI Reference Out"=w435:refnum<k20>)  [unwired: 1 in, 1 out]
                        }
                        frame #1 {
                          n160 = xnode "Read/Write Control"("FPGA VI Reference In"=w447, "FPGA Tick Reset"=FALSE, "Trigger Experiment"=TRUE ("FPGA Tick Reset")) -> ()  [unwired: 1 in, 2 out]
                        }
                      }
                    }
                    frame "409" {
                      # "flushFIFOs"
                      n161 = flat-sequence {
                        tunnel: [w451] -> w448
                        tunnel: w448 -> [w461]
                        frame #0 {
                          w454 = FALSE ("Load Actions")
                          n162 = local read "FPGA VI Reference Out"() -> (w460:refnum<k20>)
                          n163 = xnode "Read/Write Control"("FPGA VI Reference In"=w460, "Flush FIFO"=TRUE, "Load Actions Analogue 0"=w454, "Load Actions Analogue 1"=w454, "Load Actions Analogue 2"=w454, "Load Actions Digital 0"=w454) -> ("FPGA VI Reference Out"=w458:refnum<k20>)  [unwired: 1 in, 1 out]
                          n164 = xnode "Invoke Method"("FPGA VI Reference In"=w458) -> ("FPGA VI Reference Out"=w457:refnum<k20>)  [unwired: 1 in, 1 out]
                          n165 = xnode "Invoke Method"("FPGA VI Reference In"=w457) -> ("FPGA VI Reference Out"=w456:refnum<k20>)  [unwired: 1 in, 1 out]
                          n166 = xnode "Invoke Method"("FPGA VI Reference In"=w456) -> ("FPGA VI Reference Out"=w455:refnum<k20>)  [unwired: 1 in, 1 out]
                          n167 = xnode "Invoke Method"("FPGA VI Reference In"=w455) -> ("FPGA VI Reference Out"=w453:refnum<k20>)  [unwired: 1 in, 1 out]
                          n168 = xnode "Invoke Method"("FPGA VI Reference In"=w453) -> ("FPGA VI Reference Out"=w452:refnum<k20>)  [unwired: 1 in, 1 out]
                          n169 = xnode "Invoke Method"("FPGA VI Reference In"=w452) -> ("FPGA VI Reference Out"=w451:refnum<k20>)  [unwired: 1 in, 1 out]
                        }
                        frame #1 {
                          n170 = while {
                            tunnel: w461 -> [w464]
                            stop <- w462 stop-if-true
                            # "wait until FPGA target flushes FIFO"
                            n171 = xnode "Read/Write Control"("FPGA VI Reference In"=w464) -> ("Flush FIFO"=w463:bool)  [unwired: 1 in, 2 out]
                            n172 = Not(x=w463) -> (.not. x?=w462:bool)
                          }
                        }
                      }
                    }
                    frame "410" {
                      # "Digital 0, 1, 2 must be of type U32. This is because the actions are associated with a time stamp"
                      # "writeDigitals"
                      n173 = TCP Read(connection ID=w486, bytes to read=w483, 7:T5."Buffered" ("mode (standard)"), 9:-1 ("timeout ms (25000)")) -> (connection ID out=w485:refnum<k5>, data out=w481:string)  [unwired: 1 in, 1 out]
                      n174 = local read "FPGA VI Reference Out"() -> (w478:refnum<k20>)
                      n175 = Decimal String To Number(string=w481, default (0L)=u32 0 ("default (0 I32)")) -> (number=w479:u32)  [unwired: 1 in, 1 out]
                      n176 = Number To Boolean Array(number=w479) -> (Boolean array=w465:bool[])
                      "Boolean array on Host" <- w465
                      n177 = Index Array(array=w465, index=0) -> (element=w476:bool)
                      n178 = Index Array(array=w465, index=1) -> (element=w473:bool)
                      n179 = Index Array(array=w465, index=2) -> (element=w471:bool)
                      n180 = Boolean To (0,1)(Boolean=w476) -> (0, 1=w475:i16)
                      n181 = Boolean To (0,1)(Boolean=w473) -> (0, 1=w472:i16)
                      n182 = Boolean To (0,1)(Boolean=w471) -> (0, 1=w470:i16)
                      n183 = To Unsigned Long Integer(number=w475) -> (unsigned 32bit integer=w474:u32)
                      n184 = To Unsigned Long Integer(number=w472) -> (unsigned 32bit integer=w469:u32)
                      n185 = To Unsigned Long Integer(number=w470) -> (unsigned 32bit integer=w468:u32)
                      n186 = xnode "Read/Write Control"("FPGA VI Reference In"=w478, "Digital 0"=w474, "Digital 1"=w469, "Digital 2"=w468) -> ()  [unwired: 1 in, 2 out]
                    }
                    frame "411" {
                      # "writeAnalogue"
                      n187 = TCP Read(connection ID=w501, bytes to read=w497, 7:T5."Buffered" ("mode (standard)"), 9:-1 ("timeout ms (25000)")) -> (connection ID out=w498:refnum<k5>, data out=w503:string, error out=w495:errorcluster)  [unwired: 1 in]
                      n188 = Decimal String To Number(string=w503, default (0L)=u32 0 ("default (0 I32)")) -> (number=w491:u32)  [unwired: 1 in, 1 out]
                      n189 = local read "FPGA VI Reference Out"() -> (w488:refnum<k20>)
                      n190 = TCP Read(connection ID=w498, bytes to read=w497, error in (no error)=w495, 7:T5."Buffered" ("mode (standard)"), 9:-1 ("timeout ms (25000)")) -> (connection ID out=w492:refnum<k5>, data out=w493:string)  [unwired: 1 out]
                      n191 = Decimal String To Number(string=w493, default (0L)=u32 0 ("default (0 I32)")) -> (number=w489:u32)  [unwired: 1 in, 1 out]
                      n192 = case shown="Default" w491 {
                        tunnel: w489 -> [w505 w507 w509 w510 w511 _ w512]
                        tunnel: w488 -> [w506 w508 _ _ _ _ w513]
                        frame 1 {
                          n193 = xnode "Read/Write Control"("FPGA VI Reference In"=w506, "Analogue 1"=w505) -> ()  [unwired: 1 in, 2 out]
                        }
                        frame 2 {
                          n194 = xnode "Read/Write Control"("FPGA VI Reference In"=w508, "Analogue 2"=w507) -> ()  [unwired: 1 in, 2 out]
                        }
                        frame 3 {
                          n195 = local write "Analogue Line 3"(w509) -> ()
                        }
                        frame 4 {
                          n196 = local write "Analogue Line 4"(w510) -> ()
                        }
                        frame 5 {
                          n197 = local write "Analogue Line 5"(w511) -> ()
                        }
                        frame Default {
                        }
                        frame 0 {
                          n198 = xnode "Read/Write Control"("FPGA VI Reference In"=w513, "Analogue 0"=w512) -> ()  [unwired: 1 in, 2 out]
                        }
                      }
                    }
                    frame "413" {
                      # "runSequence"
                    }
                    frame "666", Default {
                    }
                  }
                  "Abort" <- w142
                }
                frame Error {
                }
              }
              n199 = call <vilib>:"General Error Handler.vi"("error in (no error)"=w123, "[exception action] (none:0)"=w125, "[exception code]"=-375005) -> ()  [unwired: 8 in, 5 out]
              n200 = local read "Status"() -> (w117:string)
              n201 = Bundle(cluster=cluster{"status":string} {"status"="OK"}, "status"=w117) -> (w134:cluster{"status":string})
              n202 = Flatten To JSON "To JSON"(anything=w134) -> (JSON string=w120:string)  [unwired: 2 in, 1 out]
              "ACK sent" <- w120
              n203 = TCP Write(connection ID=w118, data in=w120, error in (no error)=w137) -> (connection ID out=w128:refnum<k5>, bytes written=→"bytes written":i32, error out=w129:errorcluster)  [unwired: 1 in]
            }
            "remote address" <- w110
            "remote port" <- w111
          }
          frame Error {
          }
        }
        n204 = local read "Stop VI"() -> (w99:bool)
      }
      n205 = while {
        tunnel: w26 -> [w92]
        tunnel: w27 -> [w91]
        tunnel: "Receive PORT" -> [w90]
        tunnel: w29 -> [w88]
        tunnel: w24 -> [w87]
        stop <- w79 stop-if-true
        # "Analog 0: Angle\nAnalog 1: Phase\nAnalog 2: Color\nAnalog 3, 4, 5: Laser Power"
        n206 = Wait (ms)(milliseconds to wait=u32 100) -> ()  [unwired: 1 out]
        n207 = local read "Laser Toggle 0"() -> (w72:bool)
        n208 = local read "Laser Toggle 2"() -> (w70:bool)
        n209 = local read "Laser Toggle 1"() -> (w71:bool)
        n210 = Bundle By Name(cluster=T3 {"Digital 2"=FALSE, "Digital 1"=FALSE, "Digital 0"=FALSE}, "Digital 0"=w72, "Digital 1"=w71, "Digital 2"=w70) -> (w69:T3)
        n211 = Cluster To Array(cluster=w69) -> (array=w68:bool[])
        n212 = local read "Analogue Line 2"() -> (w80:u8)
        n213 = local read "Analogue Line 1"() -> (w81:u8)
        n214 = local read "Analogue Line 3"() -> (w78:u32)
        n215 = local read "Analogue Line 0"() -> (w82:u8)
        n216 = local read "Analogue Line 4"() -> (w77:u32)
        n217 = local read "Analogue Line 5"() -> (w76:u32)
        n218 = Boolean Array To Number(Boolean array=w68) -> (number=w75:u32)
        n219 = To Unsigned Byte Integer(number=w75) -> (unsigned 8bit integer=w74:u8)
        n220 = local read "Event"() -> (w83:string)
        n221 = Bundle By Name(cluster=T4 {"Digitals"=0, "Analogue 0"=0, "Analogue 1"=0, "Event"="done", "Analogue 2"=0, "Analogue 3"=0, "Analogue 4"=0, "Analogue 5"=0}, "Digitals"=w74, "Analogue 0"=w82, "Analogue 1"=w81, "Analogue 2"=w80, "Event"=w83, "Analogue 3"=w78, "Analogue 4"=w77, "Analogue 5"=w76) -> (w86:T4)
        n222 = Flatten To JSON(anything=w86) -> (JSON string=w84:string)  [unwired: 2 in, 1 out]
        "UDP Sent" <- w84
        n223 = case shown="True" w87 {
          tunnel: w92 -> [_ w98]
          tunnel: w91 -> [_ w96]
          tunnel: w90 -> [_ w95]
          tunnel: w88 -> [_ w94]
          tunnel: w84 -> [_ w93]
          frame False {
          }
          frame True {
            n224 = UDP Write(address=w98, port or service name=w95, connection ID=w96, data in=w93, 8:w94, 9:-1 ("timeout ms (25000)")) -> ()  [unwired: 2 out]
          }
        }
        n225 = local read "Stop VI"() -> (w79:bool)
      }
      n226 = TCP Close Connection(connection ID=w35, error in (no error)=w34) -> (error out=w30:errorcluster)  [unwired: 1 in, 1 out]
      n227 = call <vilib>:"Simple Error Handler.vi"("error in (no error)"=w30) -> ()  [unwired: 4 in, 5 out]
    }
    frame #3 {
      n228 = local read "FPGA VI Reference Out"() -> (w524:refnum<k20>)
      n229 = xnode "Read/Write Control"("FPGA VI Reference In"=w524, "Abort"=TRUE) -> ("FPGA VI Reference Out"=w523:refnum<k20>)  [unwired: 1 in, 1 out]
    }
    frame #4 {
      n230 = xnode "Close FPGA VI Reference"("FPGA VI Reference In"=w525) -> ()  [unwired: 1 in, 1 out]
    }
  }
